vi "Begin.vi"(8 "error in":errorcluster) -> (0 "error out":errorcluster)   [LabVIEW 2015]
doc: "Called before other user functions, this VI can be used to open I/O refnums, load in file data, and do general program initialization. Notice that the <B>error out</B> terminal is simply used for data flow. Wiring it to other structures or subVIs ensures that this VI runs first."
uses:
  Addon Motor Type Def.ctl
  <vilib>/Rock Robotics/WPI/Switch/WPI_SwitchDevRef.ctl
  <vilib>/Rock Robotics/SystemInterfaces/DIO/FPGA_DIOChannel.ctl
  <vilib>/Rock Robotics/SystemInterfaces/Counter/FPGA_CounterCtrSystemIndex.ctl
  Lidar/Lidar Type Def.ctl
  <vilib>/Rock Robotics/WPI/I2C/WPI_I2CDevRef.ctl
  <vilib>/Rock Robotics/SystemInterfaces/i2clib/i2c_bus.ctl
  <vilib>/Rock Robotics/WPI/DriverStation/WPI_DriverStationRobotMode2.ctl
  Arm/Arm Settings Type Def.ctl
  Port/PortC Settings Type Def.ctl
  Detailed Motor Type Def.ctl
  <vilib>/Rock Robotics/WPI/MotorControl/WPI_MotorControlDeviceRef.ctl
  <vilib>/Rock Robotics/WPI/MotorControl/WPI_MotorControlType.ctl
  <vilib>/Rock Robotics/SystemInterfaces/DIO/FPGA_DIOPWMChannel.ctl
  <vilib>/Rock Robotics/WPI/PWM/WPI_PWMDeadband.ctl
  <vilib>/Rock Robotics/WPI/CAN/Jaguar/SubVIs/WPI_CANJaguar_ControlMode.ctl
  <vilib>/Rock Robotics/WPI/CAN/TalonSRX/WPI_CANTalonSRX_APIControlMode.ctl
  <vilib>/Rock Robotics/WPI/CAN/TalonSRX/WPI_CANTalonSRX_APIFeedbackSelect.ctl
  Robot Global Data.vi
  <vilib>/Utility/file.llb/Read Delimited Spreadsheet (DBL).vi
  Lift/TW Global.vi
  LowShooter/Implementation/Shooter Global.vi
  <vilib>/Rock Robotics/Network Tables/NT Write Number.vi
  <vilib>/Rock Robotics/WPI/MotorControl/WPI_MotorControlOpenCANTalonSRX.vi
  <vilib>/Rock Robotics/WPI/Switch/WPI_SwitchOpenLimit.vi
  Drive/Implementation/RobotDriveGlobal.vi
panel:
  in  "Addons":T1={"SwitchDevRef"={"DevStatus"={"status"=FALSE, "code"=0, "source"=""}, "DIO Channel"=enum."Invalid", "CntIndex"=enum."Invalid", "Normally Closed"=FALSE}, "LidarRef"={"I2CDevRef"={"DevStatus"={"status"=FALSE, "code"=0, "source"=""}, "Device Address"=0, "Handle"=0, "I2C Bus"=enum."Invalid"}}, "Arm Sensors"={"Front Sensor"={"DevStatus"={"status"=FALSE, "code"=0, "source"=""}, "DIO Channel"=enum."Invalid", "CntIndex"=enum."Invalid", "Normally Closed"=FALSE}, "Back Sensor"={"DevStatus"={"status"=FALSE, "code"=0, "source"=""}, "DIO Channel"=enum."Invalid", "CntIndex"=enum."Invalid", "Normally Closed"=FALSE}, "Ball Sensor"={"DevStatus"={"status"=FALSE, "code"=0, "source"=""}, "DIO Channel"=enum."Invalid", "CntIndex"=enum."Invalid", "Normally Closed"=FALSE}}} {"LidarRef"."I2CDevRef"."Device Address" format="%.0x"}
  in  "Addon Motors":T1={"SwitchDevRef"={"DevStatus"={"status"=FALSE, "code"=0, "source"=""}, "DIO Channel"=enum."Invalid", "CntIndex"=enum."Invalid", "Normally Closed"=FALSE}, "LidarRef"={"I2CDevRef"={"DevStatus"={"status"=FALSE, "code"=0, "source"=""}, "Device Address"=0, "Handle"=0, "I2C Bus"=enum."Invalid"}}, "Arm Sensors"={"Front Sensor"={"DevStatus"={"status"=FALSE, "code"=0, "source"=""}, "DIO Channel"=enum."Invalid", "CntIndex"=enum."Invalid", "Normally Closed"=FALSE}, "Back Sensor"={"DevStatus"={"status"=FALSE, "code"=0, "source"=""}, "DIO Channel"=enum."Invalid", "CntIndex"=enum."Invalid", "Normally Closed"=FALSE}, "Ball Sensor"={"DevStatus"={"status"=FALSE, "code"=0, "source"=""}, "DIO Channel"=enum."Invalid", "CntIndex"=enum."Invalid", "Normally Closed"=FALSE}}} {"LidarRef"."I2CDevRef"."Device Address" format="%.0x"}
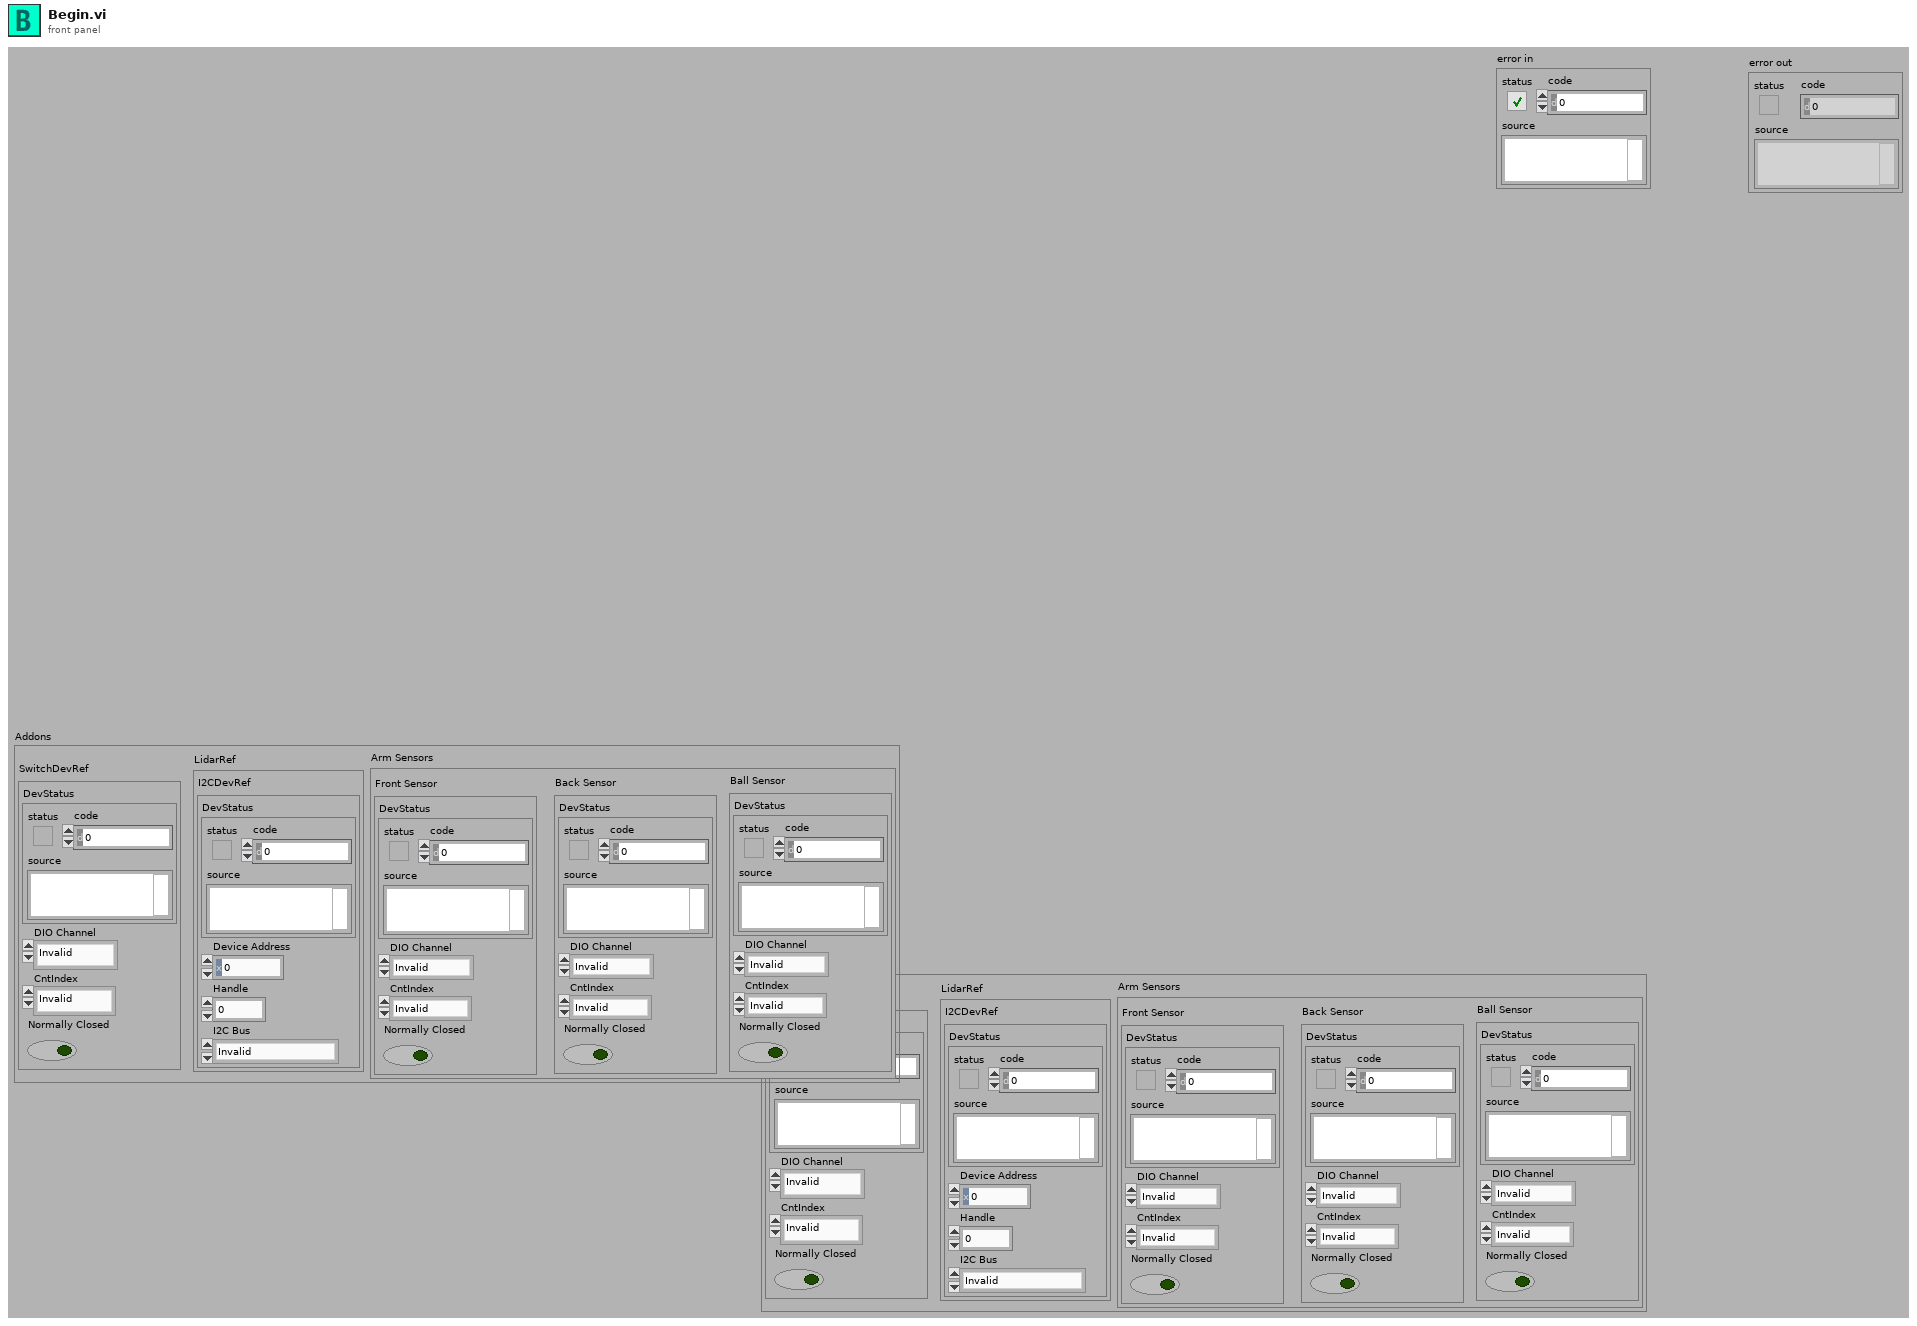
[diagram p1: front panel]
types:
  T1 = typedef "Addon Motor Type Def.ctl" = cluster{"SwitchDevRef":T2, "LidarRef":T5, "Arm Sensors":cluster{"Front Sensor":T2, "Back Sensor":T2, "Ball Sensor":T2}}
  T2 = typedef "WPI_SwitchDevRef.ctl" = cluster{"DevStatus":errorcluster, "DIO Channel":T3, "CntIndex":T4, "Normally Closed":bool}
  T3 = typedef "FPGA_DIOChannel.ctl" = enum8{"DIO 0", "DIO 1", "DIO 2", "DIO 3", "DIO 4", "DIO 5", "DIO 6", "DIO 7", "DIO 8", "DIO 9", "DIO MXP 0", "DIO MXP 1", "DIO MXP 2", "DIO MXP 3", "DIO MXP 4", "DIO MXP 5", "DIO MXP 6", "DIO MXP 7", "DIO MXP 8", "DIO MXP 9", "DIO MXP 10", "DIO MXP 11", "DIO MXP 12", "DIO MXP 13", "DIO MXP 14", "DIO MXP 15", "Invalid"}
  T4 = typedef "FPGA_CounterCtrSystemIndex.ctl" = enum8{"Ctr 0", "Ctr 1", "Ctr 2", "Ctr 3", "Ctr 4", "Ctr 5", "Ctr 6", "Ctr 7", "Invalid"}
  T5 = typedef "Lidar Type Def.ctl" = cluster{"I2CDevRef":T6}
  T6 = typedef "WPI_I2CDevRef.ctl" = cluster{"DevStatus":errorcluster, "Device Address":u8, "Handle":i32, "I2C Bus":T7}
  T7 = typedef "i2c_bus.ctl" = enum16{"I2C On-Board", "I2C MXP", "Invalid"}
  T8 = typedef "WPI_DriverStationRobotMode2.ctl" = enum16{"Autonomous Disabled", "Autonomous Enabled", "Teleop Disabled", "Teleop Enabled", "Disconnected", "Finish", "Test Disabled", "Test Enabled", "Emergency Stopped"}
  T9 = typedef "Arm Settings Type Def.ctl" = cluster{"Min Arm Pos":dbl, "Max Arm Pos":dbl, "Drive Pos":dbl, "Arm Increments":dbl, "Obstacle Pos":dbl, "Max Current":dbl}
  T10 = typedef "PortC Settings Type Def.ctl" = cluster{"Down":dbl, "Up":dbl, "Increments":dbl, "Final Pos":dbl}
  T11 = typedef "Robot Type Def.ctl" = enum32{"Disabled", "Ghost", "Casper", "Lofty", "Board", "RaceRobot", "Casper 2.0", "Excalibot 2.0"}
  T12 = typedef "Detailed Motor Type Def.ctl" = cluster{"MotorRef":T13, "Encoder Ticks Per Rev":dbl, "Set Position":dbl, "Wheel Radius":dbl}
  T13 = typedef "WPI_MotorControlDeviceRef.ctl" = cluster{"DeviceStatus":errorcluster, "Type":T14, "PWM":cluster{"PWM Channel":T15, "DeadBand":T16}, "CAN":cluster{"Device Number":u8, "Control Mode":T17, "Semaphore":T18, "Max Vout":dbl, "TalonSRX Control Mode":T19}, "Invert":bool}
  T14 = typedef "WPI_MotorControlType.ctl" = enum16{"PWM", "CAN", "CANTalonSRX"}
  T15 = typedef "FPGA_DIOPWMChannel.ctl" = enum8{"PWM 0", "PWM 1", "PWM 2", "PWM 3", "PWM 4", "PWM 5", "PWM 6", "PWM 7", "PWM 8", "PWM 9", "PWM MXP 0", "PWM MXP 1", "PWM MXP 2", "PWM MXP 3", "PWM MXP 4", "PWM MXP 5", "PWM MXP 6", "PWM MXP 7", "PWM MXP 8", "PWM MXP 9", "Invalid"}
  T16 = typedef "WPI_PWMDeadband.ctl" = cluster{"Name":string, "maxPositivePwm":i32, "minPositivePwm":i32, "centerPwm":i32, "maxNegativePwm":i32, "minNegativePwm":i32, "angularRange":u16}
  T17 = typedef "WPI_CANJaguar_ControlMode.ctl" = enum8{"Percent VBus", "Current", "Speed", "Position", "Voltage"}
  T18 = typedef "Semaphore RefNum" = refnum<k1>
  T19 = typedef "WPI_CANTalonSRX_APIControlMode.ctl" = enum8{"Percent VBus", "Speed", "Position", "Slave", "Unchanged / Invalid", "Voltage Compensation", "Current", "Motion Profile"}
  T20 = typedef "WPI_CANTalonSRX_APIFeedbackSelect.ctl" = enum16{"Digital Quadrature Encoder", "Analog Potentiometer", "Analog Encoder", "Count on Quad-A (Rising-Edge)", "Count on Quad-A (Falling-Edge)", "CTR Magnetic Enc (Absolute)", "CTR Magnetic Enc (Relative)", "Pulse Width"}
  T21 = cluster{"TW Error":errorcluster, "TWP Error":errorcluster}
  T22 = typedef "RobotDrive Type Def.ctl" = cluster{"RobotDriveDevRef":cluster{"DevStatus":errorcluster, "Motors[]":T13[], "Square Inputs":bool, "Max Output":dbl}, "Control Mode":T19, "Motor Settings":T23, "Default Control Mode":T19, "Speed Mag":dbl}
  T23 = typedef "Drive Motor Settings.ctl" = cluster{"Wheel Radius":dbl, "Encoder Ticks Per Rev":dbl, "Gear Ratio":dbl, "ClimbRev":dbl}
  T24 = typedef "JoystickMap.ctl" = cluster{"Button ID":dbl, "Joystick ID":dbl}
  T25 = typedef "WPI_JoystickDevRef.ctl" = cluster{"Device":T26}
  T26 = typedef "WPI_JoystickDeviceEnum.ctl" = enum16{"USB 0", "USB 1", "USB 2", "USB 3", "USB 4", "USB 5"}
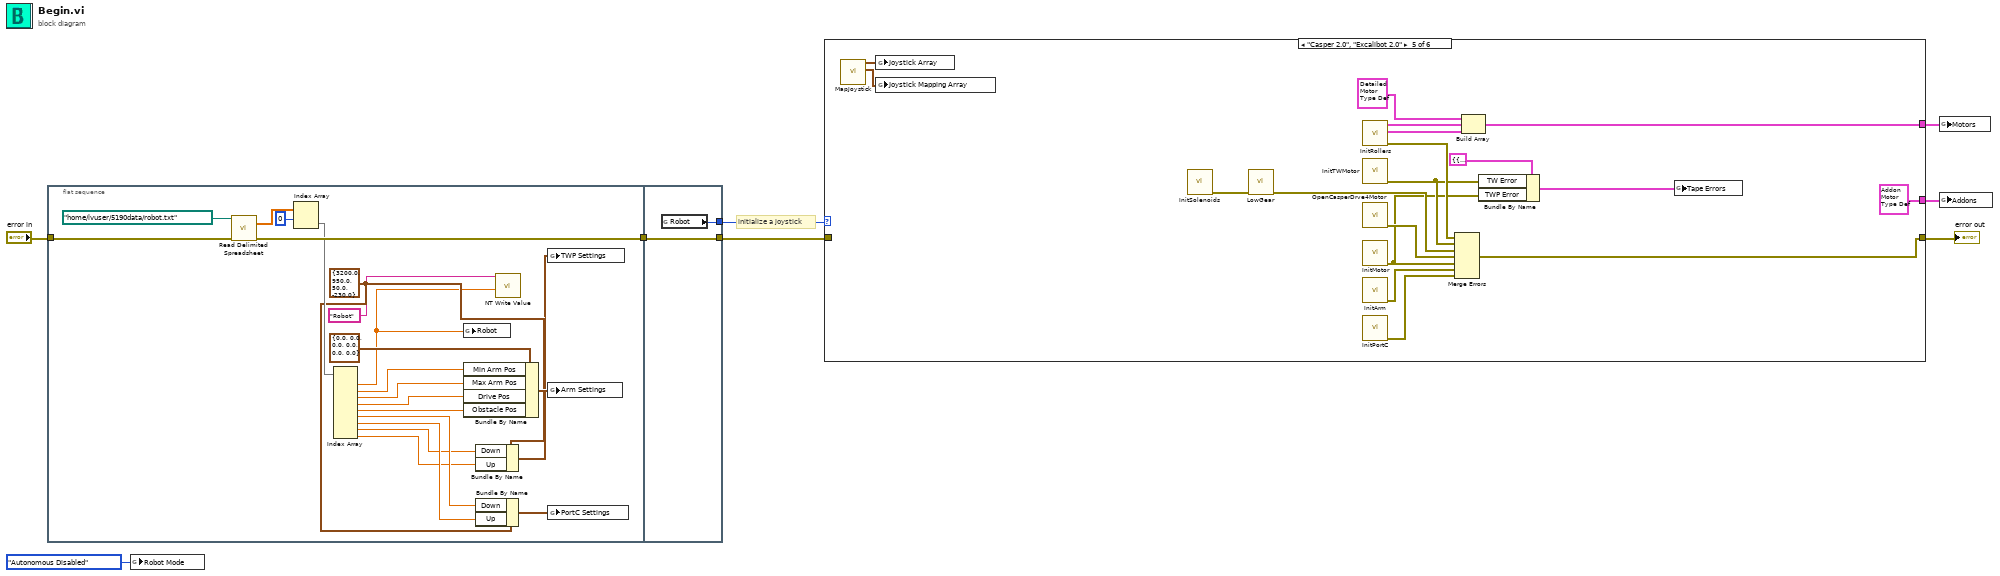
[diagram p0: block diagram]
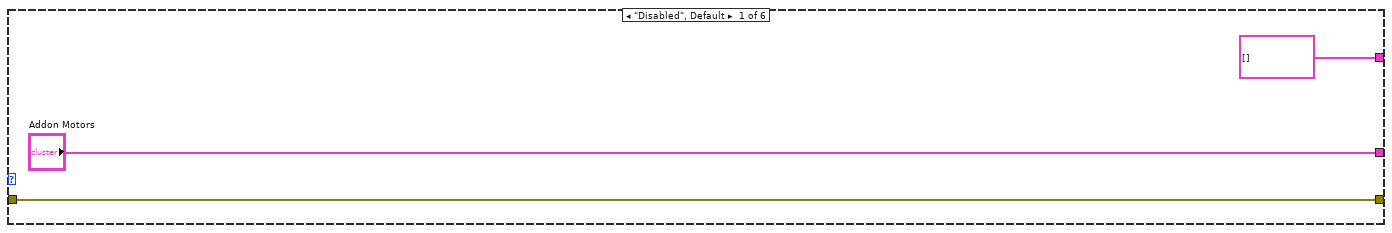
[diagram p2: hidden frame]
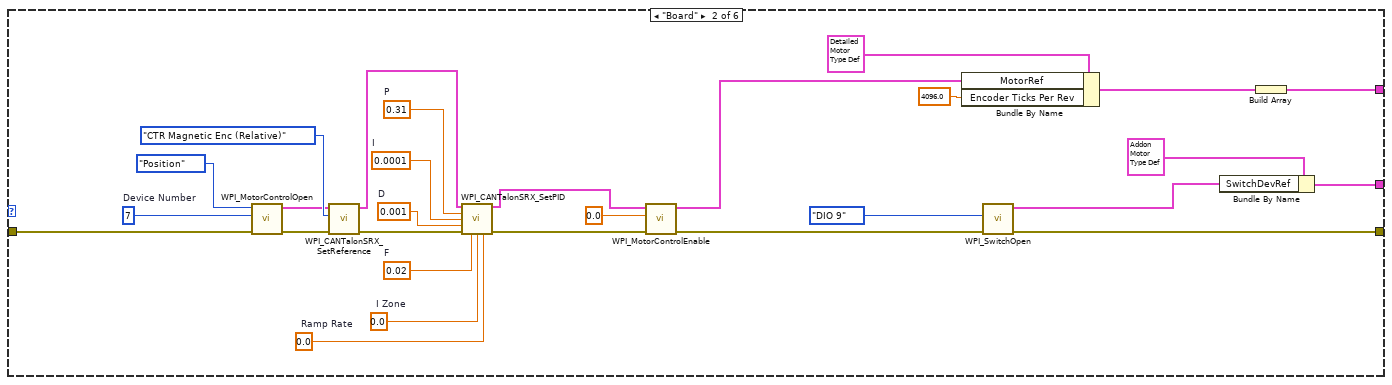
[diagram p3: hidden frame]
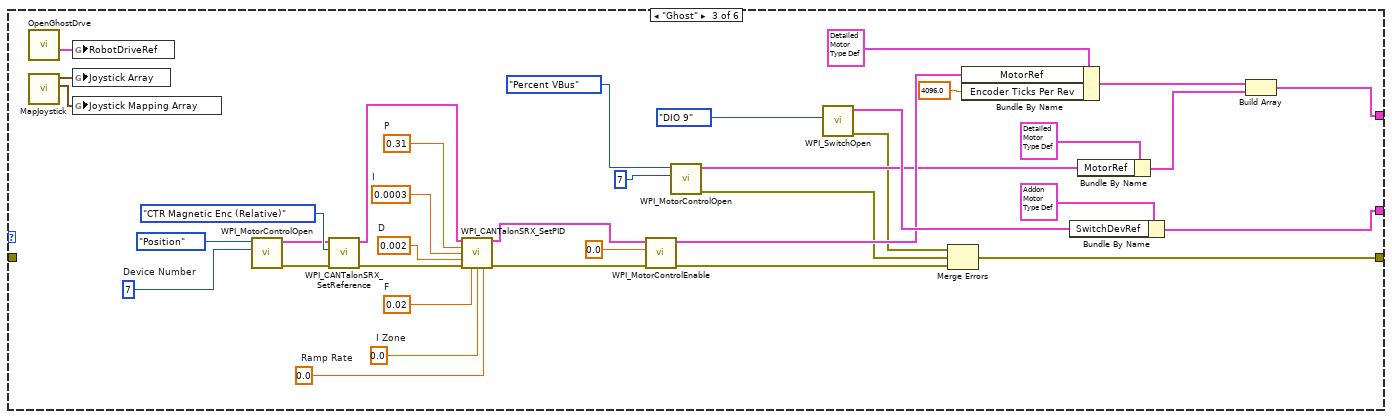
[diagram p4: hidden frame]
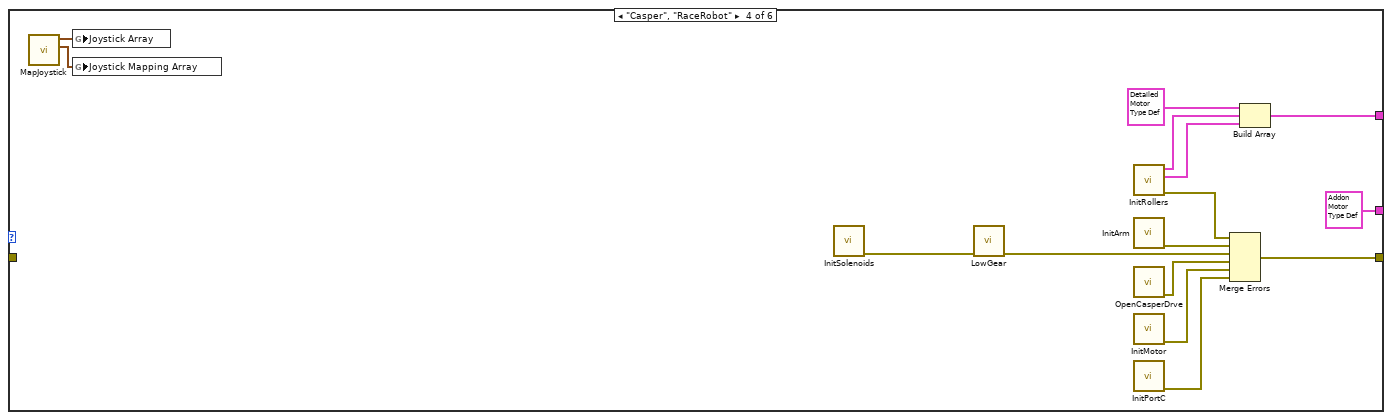
[diagram p5: hidden frame]
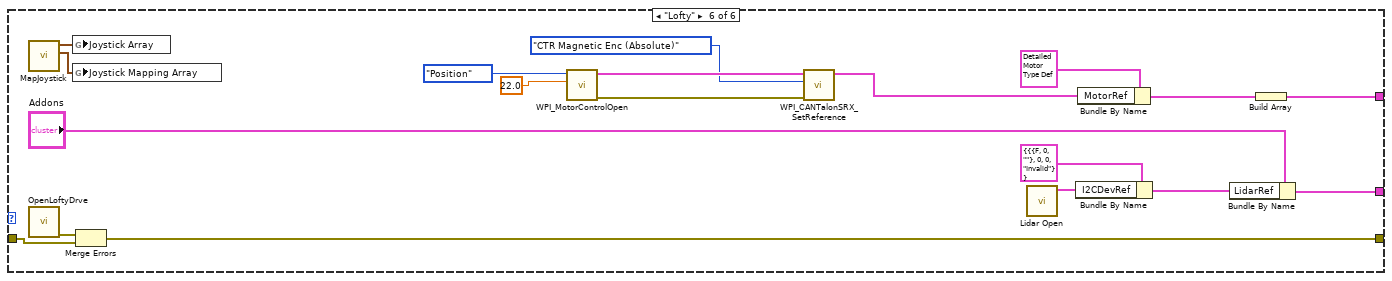
[diagram p6: hidden frame]
diagram:
  # "initialize a joystick"
  n1 = flat-sequence {
    tunnel: "error in" -> [w28]
    tunnel: [w27] -> w2
    tunnel: [w31] -> w6
    tunnel: w2 -> [w31]
    tunnel: [w30] -> w1
    frame #0 {
      w14 = T10 {"Down"=3200.0, "Up"=950.0, "Increments"=50.0, "Final Pos"=-230.0} ("PortC Settings")
      n2 = call-poly <vilib>:"Read Delimited Spreadsheet.vi"("file path (dialog if empty)"=path "/home/lvuser/5190data/robot.txt" ("file path (use dialog)"), "error in (no error)"=w28) -> ("all rows"=w26:dbl[][], "error out"=w27:errorcluster)  [unwired: 8 in, 4 out]
      n3 = Index Array(array=w26, index (row)=0) -> (element=w24:dbl[])  [unwired: 1 in]
      n4 = Index Array(array=w24) -> (element #1=w10:dbl, element #2=w22:dbl, element #3=w21:dbl, element #4=w20:dbl, element #5=w19:dbl, element #6=w17:dbl, element #7=w16:dbl, element #8=w12:dbl, element #9=w11:dbl)  [unwired: 9 in]
      n5 = global write "Robot Global Data.vi" "Robot"(w10) -> ()
      n6 = Bundle By Name(cluster=T9 {"Min Arm Pos"=0.0, "Max Arm Pos"=0.0, "Drive Pos"=0.0, "Arm Increments"=0.0, "Obstacle Pos"=0.0, "Max Current"=0.0} ("Arm Settings"), "Min Arm Pos"=w22, "Max Arm Pos"=w21, "Drive Pos"=w20, "Obstacle Pos"=w19) -> (w18:T9)
      n7 = Bundle By Name(cluster=w14, "Down"=w12, "Up"=w11) -> (w13:T10)
      n8 = Bundle By Name(cluster=w14, "Down"=w17, "Up"=w16) -> (w15:T10)
      n9 = call-poly <vilib>:"NT Write Value.vi"("Numeric"=w10, "Name"="Robot") -> ()  [unwired: 9 in, 1 out]
      n10 = global write "TW Global.vi" "TWP Settings"(w13) -> ()
      n11 = global write "Shooter Global.vi" "Arm Settings"(w18) -> ()
      n12 = global write "Robot Global Data.vi" "PortC Settings"(w15) -> ()
    }
    frame #1 {
      n13 = global read "Robot Global Data.vi" "Robot"() -> (w30:T11)
    }
  }
  n14 = global write "Robot Global Data.vi" "Robot Mode"(WPI_DriverStationRobotMode2."Autonomous Disabled" ("Robot Mode")) -> ()
  n15 = case shown="\"Casper 2.0\", \"Excalibot 2.0\"" w1 {
    tunnel: ["Addon Motors" w41 w80 T1 {"SwitchDevRef"={"DevStatus"={"status"=FALSE, "code"=0, "source"=""}, "DIO Channel"=enum."Invalid", "CntIndex"=enum."Invalid", "Normally Closed"=FALSE}, "LidarRef"={"I2CDevRef"={"DevStatus"={"status"=FALSE, "code"=0, "source"=""}, "Device Address"=0, "Handle"=0, "I2C Bus"=enum."Invalid"}}, "Arm Sensors"={"Front Sensor"={"DevStatus"={"status"=FALSE, "code"=0, "source"=""}, "DIO Channel"=enum."Invalid", "CntIndex"=enum."Invalid", "Normally Closed"=FALSE}, "Back Sensor"={"DevStatus"={"status"=FALSE, "code"=0, "source"=""}, "DIO Channel"=enum."Invalid", "CntIndex"=enum."Invalid", "Normally Closed"=FALSE}, "Ball Sensor"={"DevStatus"={"status"=FALSE, "code"=0, "source"=""}, "DIO Channel"=enum."Invalid", "CntIndex"=enum."Invalid", "Normally Closed"=FALSE}}} ("Addon Motors") T1 {"SwitchDevRef"={"DevStatus"={"status"=FALSE, "code"=0, "source"=""}, "DIO Channel"=enum."Invalid", "CntIndex"=enum."Invalid", "Normally Closed"=FALSE}, "LidarRef"={"I2CDevRef"={"DevStatus"={"status"=FALSE, "code"=0, "source"=""}, "Device Address"=0, "Handle"=0, "I2C Bus"=enum."Invalid"}}, "Arm Sensors"={"Front Sensor"={"DevStatus"={"status"=FALSE, "code"=0, "source"=""}, "DIO Channel"=enum."Invalid", "CntIndex"=enum."Invalid", "Normally Closed"=FALSE}, "Back Sensor"={"DevStatus"={"status"=FALSE, "code"=0, "source"=""}, "DIO Channel"=enum."Invalid", "CntIndex"=enum."Invalid", "Normally Closed"=FALSE}, "Ball Sensor"={"DevStatus"={"status"=FALSE, "code"=0, "source"=""}, "DIO Channel"=enum."Invalid", "CntIndex"=enum."Invalid", "Normally Closed"=FALSE}}} ("Addon Motors") w150] -> w5
    tunnel: [T12[] [] w43 w81 w114 w132 w133] -> w4
    tunnel: w6 -> [w32 w40 _ _ _ w145]
    tunnel: [w32 w35 w66 w110 w126 w144] -> w3
    frame "Disabled", Default {
    }
    frame "Board" {
      w50 = 0.0  # Ramp Rate
      w51 = 0.0  # I Zone
      w52 = 0.02  # F
      w53 = 0.001  # D
      w54 = 0.0001  # I
      w55 = 0.31  # P
      w61 = u8 7  # Device Number
      n16 = call-poly <vilib>:"WPI_MotorControlOpen.vi"("error in (no error)"=w40, "Device Number"=w61, "Control Mode"=WPI_CANTalonSRX_APIControlMode."Position") -> ("error out"=w39:errorcluster, "MotorControlDeviceRef"=w58:T13)  [unwired: 7 in]
      n17 = call <vilib>:"WPI_CANTalonSRX_SetReference.vi"("error in (no error)"=w39, "Feedback Reference"=WPI_CANTalonSRX_APIFeedbackSelect."CTR Magnetic Enc (Relative)", "CAN Talon SRX Ref"=w58) -> ("error out"=w38:errorcluster, "CAN Talon SRX Ref"=w56:T13)  [unwired: 7 in]
      n18 = call <vilib>:"WPI_CANTalonSRX_SetPID.vi"("CAN Talon SRX Ref"=w56, "P"=w55, "I"=w54, "D"=w53, "error in (no error)"=w38, "F"=w52, "I Zone"=w51, "Ramp Rate"=w50) -> ("CAN Talon SRX Ref"=w57:T13, "error out"=w37:errorcluster)  [unwired: 6 in]
      n19 = call <vilib>:"WPI_MotorControlEnable.vi"("error in (no error)"=w37, "Encoder Initial Position"=0.0, "CAN MotorDevRef"=w57) -> ("error out"=w36:errorcluster, "CAN MotorDevRef"=w48:T13)  [unwired: 7 in]
      n20 = Bundle By Name(cluster=T12 {"MotorRef"={"DeviceStatus"={"status"=FALSE, "code"=0, "source"=""}, "Type"=enum."PWM", "PWM"={"PWM Channel"=enum."Invalid", "DeadBand"={"Name"="", "maxPositivePwm"=0, "minPositivePwm"=0, "centerPwm"=0, "maxNegativePwm"=0, "minNegativePwm"=0, "angularRange"=0}}, "CAN"={"Device Number"=0, "Control Mode"=enum."Percent VBus", "Semaphore"=refnum, "Max Vout"=12.0, "TalonSRX Control Mode"=enum."Percent VBus"}, "Invert"=FALSE}, "Encoder Ticks Per Rev"=0.0, "Set Position"=0.0, "Wheel Radius"=0.0} ("Detaled Motor Type Def"), "MotorRef"=w48, "Encoder Ticks Per Rev"=4096.0) -> (w44:T12)
      n21 = call-poly <vilib>:"WPI_SwitchOpen.vi"("error in (no error)"=w36, "DIO Channel"=FPGA_DIOChannel."DIO 9") -> ("error out"=w35:errorcluster, "SwitchDevRef"=w45:T2)  [unwired: 8 in]
      n22 = Bundle By Name(cluster=T1 {"SwitchDevRef"={"DevStatus"={"status"=FALSE, "code"=0, "source"=""}, "DIO Channel"=enum."Invalid", "CntIndex"=enum."Invalid", "Normally Closed"=FALSE}, "LidarRef"={"I2CDevRef"={"DevStatus"={"status"=FALSE, "code"=0, "source"=""}, "Device Address"=0, "Handle"=0, "I2C Bus"=enum."Invalid"}}, "Arm Sensors"={"Front Sensor"={"DevStatus"={"status"=FALSE, "code"=0, "source"=""}, "DIO Channel"=enum."Invalid", "CntIndex"=enum."Invalid", "Normally Closed"=FALSE}, "Back Sensor"={"DevStatus"={"status"=FALSE, "code"=0, "source"=""}, "DIO Channel"=enum."Invalid", "CntIndex"=enum."Invalid", "Normally Closed"=FALSE}, "Ball Sensor"={"DevStatus"={"status"=FALSE, "code"=0, "source"=""}, "DIO Channel"=enum."Invalid", "CntIndex"=enum."Invalid", "Normally Closed"=FALSE}}} ("Addon Motors"), "SwitchDevRef"=w45) -> (w41:T1)
      n23 = Build Array(w44) -> (w43:T12[])
    }
    frame "Ghost" {
      w85 = 0.0  # Ramp Rate
      w86 = 0.0  # I Zone
      w87 = 0.02  # F
      w88 = 0.002  # D
      w89 = 0.0003  # I
      w90 = 0.31  # P
      w96 = u8 7  # Device Number
      n24 = call "OpenGhostDrve.vi"() -> ("RobotDriveRef"=w69:T22)  [unwired: 9 in, 2 out]
      n25 = call "MapJoystick.vi"() -> ("Joystick Map"=w68:T24[], "Joysticks"=w67:T25[])  [unwired: 10 in]
      n26 = global write "RobotDriveGlobal.vi" "RobotDriveRef"(w69) -> ()
      n27 = global write "Robot Global Data.vi" "Joystick Array"(w67) -> ()
      n28 = global write "Robot Global Data.vi" "Joystick Mapping Array"(w68) -> ()
      n29 = call-poly <vilib>:"WPI_MotorControlOpen.vi"("Device Number"=w96, "Control Mode"=WPI_CANTalonSRX_APIControlMode."Position") -> ("error out"=w78:errorcluster, "MotorControlDeviceRef"=w93:T13)  [unwired: 8 in]
      n30 = call <vilib>:"WPI_CANTalonSRX_SetReference.vi"("error in (no error)"=w78, "Feedback Reference"=WPI_CANTalonSRX_APIFeedbackSelect."CTR Magnetic Enc (Relative)", "CAN Talon SRX Ref"=w93) -> ("error out"=w77:errorcluster, "CAN Talon SRX Ref"=w91:T13)  [unwired: 7 in]
      n31 = call <vilib>:"WPI_CANTalonSRX_SetPID.vi"("CAN Talon SRX Ref"=w91, "P"=w90, "I"=w89, "D"=w88, "error in (no error)"=w77, "F"=w87, "I Zone"=w86, "Ramp Rate"=w85) -> ("CAN Talon SRX Ref"=w92:T13, "error out"=w76:errorcluster)  [unwired: 6 in]
      n32 = call <vilib>:"WPI_MotorControlEnable.vi"("error in (no error)"=w76, "Encoder Initial Position"=0.0, "CAN MotorDevRef"=w92) -> ("error out"=w63:errorcluster, "CAN MotorDevRef"=w84:T13)  [unwired: 7 in]
      n33 = call-poly <vilib>:"WPI_MotorControlOpen.vi"("Device Number"=u8 7, "Control Mode"=WPI_CANTalonSRX_APIControlMode."Percent VBus") -> ("error out"=w64:errorcluster, "MotorControlDeviceRef"=w72:T13)  [unwired: 8 in]
      n34 = call-poly <vilib>:"WPI_SwitchOpen.vi"("DIO Channel"=FPGA_DIOChannel."DIO 9") -> ("error out"=w65:errorcluster, "SwitchDevRef"=w98:T2)  [unwired: 9 in]
      n35 = Merge Errors(w65, w64, w63) -> (w66:errorcluster)
      n36 = Bundle By Name(cluster=T12 {"MotorRef"={"DeviceStatus"={"status"=FALSE, "code"=0, "source"=""}, "Type"=enum."PWM", "PWM"={"PWM Channel"=enum."Invalid", "DeadBand"={"Name"="", "maxPositivePwm"=0, "minPositivePwm"=0, "centerPwm"=0, "maxNegativePwm"=0, "minNegativePwm"=0, "angularRange"=0}}, "CAN"={"Device Number"=0, "Control Mode"=enum."Percent VBus", "Semaphore"=refnum, "Max Vout"=12.0, "TalonSRX Control Mode"=enum."Percent VBus"}, "Invert"=FALSE}, "Encoder Ticks Per Rev"=0.0, "Set Position"=0.0, "Wheel Radius"=0.0} ("Detaled Motor Type Def"), "MotorRef"=w84, "Encoder Ticks Per Rev"=4096.0) -> (w82:T12)
      n37 = Bundle By Name(cluster=T1 {"SwitchDevRef"={"DevStatus"={"status"=FALSE, "code"=0, "source"=""}, "DIO Channel"=enum."Invalid", "CntIndex"=enum."Invalid", "Normally Closed"=FALSE}, "LidarRef"={"I2CDevRef"={"DevStatus"={"status"=FALSE, "code"=0, "source"=""}, "Device Address"=0, "Handle"=0, "I2C Bus"=enum."Invalid"}}, "Arm Sensors"={"Front Sensor"={"DevStatus"={"status"=FALSE, "code"=0, "source"=""}, "DIO Channel"=enum."Invalid", "CntIndex"=enum."Invalid", "Normally Closed"=FALSE}, "Back Sensor"={"DevStatus"={"status"=FALSE, "code"=0, "source"=""}, "DIO Channel"=enum."Invalid", "CntIndex"=enum."Invalid", "Normally Closed"=FALSE}, "Ball Sensor"={"DevStatus"={"status"=FALSE, "code"=0, "source"=""}, "DIO Channel"=enum."Invalid", "CntIndex"=enum."Invalid", "Normally Closed"=FALSE}}} ("Addon Motors"), "SwitchDevRef"=w98) -> (w80:T1)
      n38 = Bundle By Name(cluster=T12 {"MotorRef"={"DeviceStatus"={"status"=FALSE, "code"=0, "source"=""}, "Type"=enum."PWM", "PWM"={"PWM Channel"=enum."Invalid", "DeadBand"={"Name"="", "maxPositivePwm"=0, "minPositivePwm"=0, "centerPwm"=0, "maxNegativePwm"=0, "minNegativePwm"=0, "angularRange"=0}}, "CAN"={"Device Number"=0, "Control Mode"=enum."Percent VBus", "Semaphore"=refnum, "Max Vout"=12.0, "TalonSRX Control Mode"=enum."Percent VBus"}, "Invert"=FALSE}, "Encoder Ticks Per Rev"=0.0, "Set Position"=0.0, "Wheel Radius"=0.0} ("Detaled Motor Type Def"), "MotorRef"=w72) -> (w71:T12)
      n39 = Build Array(w82, w71) -> (w81:T12[])
    }
    frame "Casper", "RaceRobot" {
      n40 = call "MapJoystick.vi"() -> ("Joystick Map"=w109:T24[], "Joysticks"=w108:T25[])  [unwired: 10 in]
      n41 = global write "Robot Global Data.vi" "Joystick Array"(w108) -> ()
      n42 = global write "Robot Global Data.vi" "Joystick Mapping Array"(w109) -> ()
      n43 = call "InitSolenoids.vi"() -> ("error out"=w101:errorcluster)  [unwired: 11 in]
      n44 = call "LowGear.vi"("error in (no error)"=w101) -> ("error out"=w100:errorcluster)  [unwired: 10 in]
      n45 = call "InitRollers.vi"() -> ("error out"=w102:errorcluster, "Top Roller"=w112:T12, "Bottom Roller"=w113:T12)  [unwired: 9 in]
      n46 = call "InitArm.vi"() -> ("error out"=w104:errorcluster)  [unwired: 11 in]
      n47 = call "OpenCasperDrve.vi"() -> ("error out"=w111:errorcluster)  [unwired: 10 in, 1 out]
      n48 = call "InitMotor.vi"() -> ("error out"=w107:errorcluster)  [unwired: 11 in]
      n49 = call "InitPortC.vi"() -> ("error out"=w103:errorcluster)  [unwired: 10 in, 1 out]
      n50 = Merge Errors(w102, w104, w100, w111, w107, w103) -> (w110:errorcluster)
      n51 = Build Array(T12 {"MotorRef"={"DeviceStatus"={"status"=FALSE, "code"=0, "source"=""}, "Type"=enum."PWM", "PWM"={"PWM Channel"=enum."Invalid", "DeadBand"={"Name"="", "maxPositivePwm"=0, "minPositivePwm"=0, "centerPwm"=0, "maxNegativePwm"=0, "minNegativePwm"=0, "angularRange"=0}}, "CAN"={"Device Number"=0, "Control Mode"=enum."Percent VBus", "Semaphore"=refnum, "Max Vout"=12.0, "TalonSRX Control Mode"=enum."Percent VBus"}, "Invert"=FALSE}, "Encoder Ticks Per Rev"=0.0, "Set Position"=0.0, "Wheel Radius"=0.0} ("Detaled Motor Type Def"), w113, w112) -> (w114:T12[])
    }
    frame "Casper 2.0", "Excalibot 2.0" {
      n52 = call "MapJoystick.vi"() -> ("Joystick Map"=w131:T24[], "Joysticks"=w130:T25[])  [unwired: 10 in]
      n53 = global write "Robot Global Data.vi" "Joystick Array"(w130) -> ()
      n54 = global write "Robot Global Data.vi" "Joystick Mapping Array"(w131) -> ()
      n55 = call "InitSolenoids.vi"() -> ("error out"=w125:errorcluster)  [unwired: 11 in]
      n56 = call "LowGear.vi"("error in (no error)"=w125) -> ("error out"=w124:errorcluster)  [unwired: 10 in]
      n57 = call "InitRollers.vi"() -> ("error out"=w121:errorcluster, "Top Roller"=w122:T12, "Bottom Roller"=w123:T12)  [unwired: 9 in]
      n58 = call "InitTWMotor.vi"() -> ("error out"=w116:errorcluster)  [unwired: 11 in]
      n59 = call "OpenCasperDrve4Motor.vi"() -> ("error out"=w127:errorcluster)  [unwired: 10 in, 1 out]
      n60 = call "InitMotor.vi"() -> ("error out"=w115:errorcluster)  [unwired: 11 in]
      n61 = call "InitArm.vi"() -> ("error out"=w120:errorcluster)  [unwired: 11 in]
      n62 = call "InitPortC.vi"() -> ("error out"=w119:errorcluster)  [unwired: 10 in, 1 out]
      n63 = Merge Errors(w121, w116, w124, w127, w115, w120, w119) -> (w126:errorcluster)
      n64 = Build Array(T12 {"MotorRef"={"DeviceStatus"={"status"=FALSE, "code"=0, "source"=""}, "Type"=enum."PWM", "PWM"={"PWM Channel"=enum."Invalid", "DeadBand"={"Name"="", "maxPositivePwm"=0, "minPositivePwm"=0, "centerPwm"=0, "maxNegativePwm"=0, "minNegativePwm"=0, "angularRange"=0}}, "CAN"={"Device Number"=0, "Control Mode"=enum."Percent VBus", "Semaphore"=refnum, "Max Vout"=12.0, "TalonSRX Control Mode"=enum."Percent VBus"}, "Invert"=FALSE}, "Encoder Ticks Per Rev"=0.0, "Set Position"=0.0, "Wheel Radius"=0.0} ("Detaled Motor Type Def"), w123, w122) -> (w132:T12[])
      n65 = Bundle By Name(cluster=T21 {"TW Error"={"status"=FALSE, "code"=0, "source"=""}, "TWP Error"={"status"=FALSE, "code"=0, "source"=""}} ("Tape Errors"), "TW Error"=w116, "TWP Error"=w115) -> (w118:T21)
      n66 = global write "TW Global.vi" "Tape Errors"(w118) -> ()
    }
    frame "Lofty" {
      n67 = call "MapJoystick.vi"() -> ("Joystick Map"=w143:T24[], "Joysticks"=w142:T25[])  [unwired: 10 in]
      n68 = call "OpenLoftyDrve.vi"() -> ("error out"=w146:errorcluster)  [unwired: 11 in]
      n69 = global write "Robot Global Data.vi" "Joystick Array"(w142) -> ()
      n70 = global write "Robot Global Data.vi" "Joystick Mapping Array"(w143) -> ()
      n71 = Merge Errors(w146, w145) -> (w144:errorcluster)
      n72 = call-poly <vilib>:"WPI_MotorControlOpen.vi"("Device Number"=22.0 ("New Sensor Position"), "Control Mode"=WPI_CANTalonSRX_APIControlMode."Position") -> ("error out"=w138:errorcluster, "MotorControlDeviceRef"=w139:T13)  [unwired: 8 in]
      n73 = call <vilib>:"WPI_CANTalonSRX_SetReference.vi"("error in (no error)"=w138, "Feedback Reference"=WPI_CANTalonSRX_APIFeedbackSelect."CTR Magnetic Enc (Absolute)", "CAN Talon SRX Ref"=w139) -> ("CAN Talon SRX Ref"=w135:T13)  [unwired: 7 in, 1 out]
      n74 = call "Lidar Open.vi"() -> ("I2CDevRef"=w148:T6)  [unwired: 11 in]
      n75 = Bundle By Name(cluster=T5 {"I2CDevRef"={"DevStatus"={"status"=FALSE, "code"=0, "source"=""}, "Device Address"=0, "Handle"=0, "I2C Bus"=enum."Invalid"}} ("LidarRef"), "I2CDevRef"=w148) -> (w147:T5)
      n76 = Bundle By Name(cluster=T12 {"MotorRef"={"DeviceStatus"={"status"=FALSE, "code"=0, "source"=""}, "Type"=enum."PWM", "PWM"={"PWM Channel"=enum."Invalid", "DeadBand"={"Name"="", "maxPositivePwm"=0, "minPositivePwm"=0, "centerPwm"=0, "maxNegativePwm"=0, "minNegativePwm"=0, "angularRange"=0}}, "CAN"={"Device Number"=0, "Control Mode"=enum."Percent VBus", "Semaphore"=refnum, "Max Vout"=12.0, "TalonSRX Control Mode"=enum."Percent VBus"}, "Invert"=FALSE}, "Encoder Ticks Per Rev"=0.0, "Set Position"=0.0, "Wheel Radius"=0.0} ("Detaled Motor Type Def"), "MotorRef"=w135) -> (w134:T12)
      n77 = Bundle By Name(cluster="Addons", "LidarRef"=w147) -> (w150:T1)
      n78 = Build Array(w134) -> (w133:T12[])
    }
  }
  "error out" <- w3
  n79 = global write "Robot Global Data.vi" "Motors"(w4) -> ()
  n80 = global write "Robot Global Data.vi" "Addons"(w5) -> ()
